vi "Temperature Engine Driver.vi"(11 "Sequence":refnum<k7>) -> (0 "error out":errorcluster)   [LabVIEW 2023, in "LTT_TeststandSteptypes.lvlib"]
uses:
  LTT_TeststandSteptypes.lvlib
  HardwareAbstractionLayer_LVOOP/Modbus/Modbus_class/Modbus.lvclass
  HardwareAbstractionLayer_LVOOP/Report/Report_class/Control/Temperature LOG.ctl
  Control/TC FGV Action.ctl
  HardwareAbstractionLayer_LVOOP/Power Moniter/Wait Monitor_class/SubVI/Control/TimerStates.ctl
  HardwareAbstractionLayer_LVOOP/Report/Report_class/Control/All Log Details.ctl
  HardwareAbstractionLayer_LVOOP/Report/Report_class/Control/UUT Test Info.ctl
  HardwareAbstractionLayer_LVOOP/Report/Report_class/Control/FE FRAME LOG.ctl
  HardwareAbstractionLayer_LVOOP/Report/Report_class/Control/FF FRAME LOG.ctl
  HardwareAbstractionLayer_LVOOP/Report/Report_class/Control/LIMIT TABLE.ctl
  HardwareAbstractionLayer_LVOOP/Report/Report_class/Control/ERROR LOG APPEND.ctl
  HardwareAbstractionLayer_LVOOP/Report/Report_class/Control/ERROR LOG.ctl
  HardwareAbstractionLayer_LVOOP/Report/Report_class/Control/FA FRAME LOG.ctl
  HardwareAbstractionLayer_LVOOP/Report/Report_class/Control/TEST RESULT LOG APPEND.ctl
  HardwareAbstractionLayer_LVOOP/Report/Report_class/Control/TEST RESULT LOG.ctl
  HardwareAbstractionLayer_LVOOP/Report/Report_class/Control/SYSTEM LOG.ctl
  HardwareAbstractionLayer_LVOOP/Report/Report_class/Control/POWER STATUS.ctl
  HardwareAbstractionLayer_LVOOP/Report/Report_class/Control/CYCLE_DURATION_LOG.ctl
  99722fe1-a764-4b52-b67b-c7e93846cf84.vi
  930c386e-a8bd-4bc2-a3c6-04cbbef34728.vi
  767a7da0-b67a-495a-b36e-4f64d8e2d20e.vi
  <vilib>/addons/TestStand/_TSUtility.llb/TestStand - Get Property Value (Boolean).vi
  GlobalVariable/GlobalVariableData.vi
  <vilib>/addons/TestStand/_TSUtility.llb/TestStand - Get Property Value (Number {Unsigned 32-bit Integer}).vi
  <vilib>/addons/TestStand/_TSUtility.llb/TestStand - Set Property Value (Number {Signed 16-bit Integer}).vi
  <vilib>/addons/TestStand/_TSUtility.llb/TestStand - Set Property Value (Boolean).vi
  <vilib>/addons/TestStand/_TSUtility.llb/TestStand - Set Property Value (String).vi
  HardwareAbstractionLayer_LVOOP/Database/Database.lvclass
  HardwareAbstractionLayer_LVOOP/Database/SQL Public VI/Control/DB Options.ctl
  HardwareAbstractionLayer_LVOOP/Teststand/Teststand.lvclass
  HardwareAbstractionLayer_LVOOP/Power Moniter/Wait Monitor_class/Wait Monitor.lvclass
  HardwareAbstractionLayer_LVOOP/Report/Report_class/Report.lvclass
panel:
  out "Array":i32[](array[numeric])
  out "End":string
  in  "Stop":bool
  in  "Modbus RTU":T1={"unit ID"=1, "serial type"=enum."RTU", "baud rate"=9600, "parity (even)"=2, "flow control (none)"=0, "VISA resource name"=""} {"flow control (none)" items=["None", "XON/XOFF", "RTS/CTS", "XON/XOFF & RTS/CTS", "DTR/DSR", "XON/XOFF & DTR/DSR"]; "parity (even)" items=["None", "Odd", "Even", "Mark", "Space"]}
  in  "error in":errorcluster
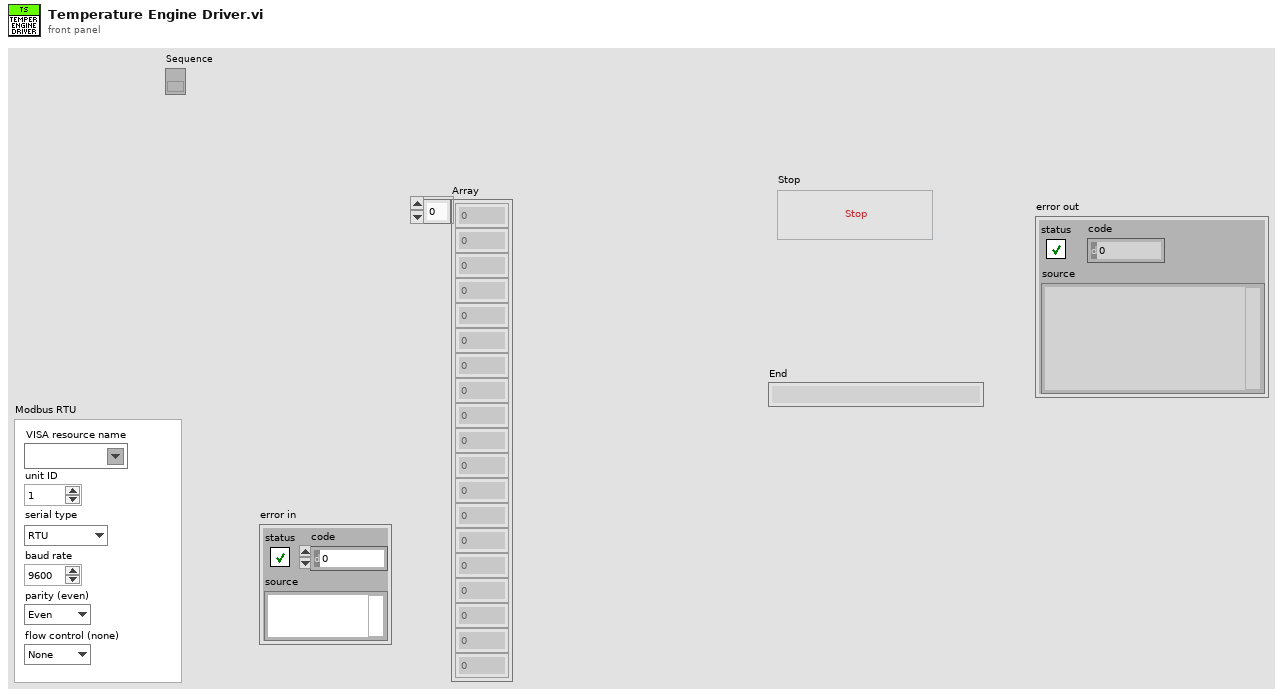
[diagram p1: front panel]
types:
  T1 = cluster{"unit ID":u8, "serial type":enum16{"RTU", "ASCII"}, "baud rate":u32, "parity (even)":u16, "flow control (none)":u16, "VISA resource name":refnum<visa-resource-name>}
  T2 = typedef "HardwareAbstractionLayer_LVOOP.lvlib/Report.lvclass/Temperature LOG.ctl" = cluster{"TEST_MODE":string, "CYCLE_NUMBER":string, "TEMPERATURE":cluster{"LV_PPS_TEMPERATURE":dbl, "HV_PPS1_TEMPERATURE":dbl, "HV_PPS2_TEMPERATURE":dbl, "HV_PPS3_TEMPERATURE":dbl, "HV_PPS4_TEMPERATURE":dbl, "HV_PPS5_TEMPERATURE":dbl, "HV_PPS6_TEMPERATURE":dbl, "CHAMBER_TEMPERATURE":dbl, "LOAD_U1_TEMPERATURE":dbl, "LOAD_V1_TEMPERATURE":dbl, "LOAD_W1_TEMPERATURE":dbl, "LOAD_U2_TEMPERATURE":dbl, "LOAD_V2_TEMPERATURE":dbl, "LOAD_W2_TEMPERATURE":dbl, "LOAD_U3_TEMPERATURE":dbl, "LOAD_V3_TEMPERATURE":dbl, "LOAD_W3_TEMPERATURE":dbl}, "Temperature Inrange":cluster{"LVPPS_Trip?":bool, "HVPPS1_Trip?":bool, "HVPPS2_Trip?":bool, "HVPPS3_Trip?":bool, "HVPPS4_Trip?":bool, "HVPPS5_Trip?":bool, "HVPPS6_Trip?":bool, "Chamber_Trip?":bool}}
  T3 = typedef "HardwareAbstractionLayer_LVOOP.lvlib/Database.lvclass/DB Options.ctl" = enum16{"Init", "Select Data", "Insert Data", "Update Data", "Delete Data", "Execute Query", "Create Schema", "Create Table", "List Tables", "List Columns", "Close"}
  T4 = typedef "TestStand - Status Monitor.ctl" = cluster{"Sequence Context":refnum<k7>, "Execution":refnum<k7>, "Termination Monitor":refnum<k7>}
  T5 = typedef "HardwareAbstractionLayer_LVOOP.lvlib/Report.lvclass/All Log Details.ctl" = cluster{"UUT_TEST_INFO":T6, "FE_FRAME_LOG":T7, "FF_FRAME_LOG":T8, "LIMIT_TABLE":T9, "ERROR LOG Append":T10, "FA_FRAME_LOG":T12, "Socket No":u16, "TEST RESULT LOG Append":T13, "SYSTEM_LOG":T15, "Temperature log":T2, "POWER_STATUS":T16, "CYCLE_DURATION_LOG":T17}
  T6 = typedef "HardwareAbstractionLayer_LVOOP.lvlib/Report.lvclass/UUT Test Info.ctl" = cluster{"ID":string, "STATION_ID":string, "TEST_SOCKET_INDEX":string, "UUT_SERIAL_NUMBER":string, "TSW_VER":string, "VAL_SW_VER":string, "PROJECT_NAME":string, "PRODUCT_NAME":string, "PRODUCT_VARIANT":string, "TEST_NAME":string, "TEST_PHASE":string, "TEST_DESCRIPTION":string, "TEMP_CHAMBER_NAME":string, "START_DATE_TIME":string, "STOP_DATE_TIME ":string, "START_CYCLE_COUNT":string, "STOP_CYCLE_COUNT":string, "EXECUTION_TIME":string, "UUT_STATUS":string, "UUT_ERROR_CODE":string, "UUT_ERROR_MESSAGE":string, "TEST_SEQUENCE":string}
  T7 = typedef "HardwareAbstractionLayer_LVOOP.lvlib/Report.lvclass/FE FRAME LOG.ctl" = cluster{"ID":string, "UUT_TEST_INFO":string, "DATE_TIME":string, "CYCLE_NUMBER":string, "TEST_MODE":string, "CHAMBER_TEMP":string, "CAN_FRAME_RX":string, "Test Mode":u32, "LV_PPS_VOLTAGE":string, "LV_PPS_CURRENT":string, "HV_PPS_VOLTAGE":string, "HV_PPS_CURRENT":string, "SOCKET_NUMBER":string, "CAN_FRAME_RX_NO_OFF_BYTE":string}
  T8 = typedef "HardwareAbstractionLayer_LVOOP.lvlib/Report.lvclass/FF FRAME LOG.ctl" = cluster{"ID":string, "UUT_TEST_INFO":string, "DATE_TIME":string, "CYCLE_NUMBER":string, "TEST_MODE":string, "CAN_FRAME_RX":string, "CHAMBER_TEMP":string, "TestMode":u32, "SOCKET_NUMBER":string, "CAN_FRAME_RX_NO_OFF_BYTE":string}
  T9 = typedef "HardwareAbstractionLayer_LVOOP.lvlib/Report.lvclass/LIMIT TABLE.ctl" = cluster{"ID":string, "PRODUCT_NAME":string, "PRODUCT_VARIANT":string, "TEST_MODE":string, "PARAMETER_NAME":string, "COMPARISON_TYPE":string, "LOW_LIMIT":string, "HIGH_LIMIT":string, "UNIT":string, "ERROR_MESSSAGE":string, "SEVERITY":string}
  T10 = typedef "HardwareAbstractionLayer_LVOOP.lvlib/Report.lvclass/ERROR LOG APPEND.ctl" = T11[]
  T11 = typedef "HardwareAbstractionLayer_LVOOP.lvlib/Report.lvclass/ERROR LOG.ctl" = cluster{"ID":string, "UUT_TEST_INFO":string, "DATE_TIME":string, "CYCLE_NUMBER":string, "TEST_MODE":string, "SIGNAL_NAME":string, "SIGNAL_VALUE":string, "UNIT":string, "COMPARISON_VALUE":string, "ERROR_MESSAGE":string, "FRAME_TYPE":string, "LIMITID":string, "SOCKET_NUMBER":string}
  T12 = typedef "HardwareAbstractionLayer_LVOOP.lvlib/Report.lvclass/FA FRAME LOG.ctl" = cluster{"UUT_TEST_INFO":string, "CAN_FRAME_RX":string, "CAN_FRAME_RX_NO_OFF_BYTE":string}
  T13 = typedef "HardwareAbstractionLayer_LVOOP.lvlib/Report.lvclass/TEST RESULT LOG APPEND.ctl" = T14[]
  T14 = typedef "HardwareAbstractionLayer_LVOOP.lvlib/Report.lvclass/TEST RESULT LOG.ctl" = cluster{"ID":string, "UUT_TEST_INFO":string, "DATE_TIME":string, "CYCLE_NUMBER":string, "TEST_MODE":string, "SIGNAL_NAME":string, "SIGNAL_VALUE":string, "COMPARISON_VALUE":string, "ERROR_MESSAGE":string, "FRAME_TYPE":string, "LIMITID":string, "TEST_RESULT":string, "SOCKET_NUMBER":string}
  T15 = typedef "HardwareAbstractionLayer_LVOOP.lvlib/Report.lvclass/SYSTEM LOG.ctl" = cluster{"ID ":string, "DATE_TIME":string, "CYCLE_NUMBER":string, "TEST_MODE":string, "ERROR_MESSAGE":string}
  T16 = typedef "HardwareAbstractionLayer_LVOOP.lvlib/Report.lvclass/POWER STATUS.ctl" = cluster{"TEST_MODE":string, "CYCLE_NUMBER":string, "TYPE_POWER":string, "STATE":string}
  T17 = typedef "HardwareAbstractionLayer_LVOOP.lvlib/Report.lvclass/CYCLE_DURATION_LOG.ctl" = cluster{"CYCLE_NUMBER":string}
  T18 = typedef "HardwareAbstractionLayer_LVOOP.lvlib/Wait Monitor.lvclass/TimerStates.ctl" = enum16{"Run", "Pause", "Reset"}
  T19 = typedef "LTT_TeststandSteptypes.lvlib/TC FGV Action.ctl" = enum16{"Set", "Get"}
  T20 = cluster{"Chamber Present Temp":dbl, "Chamber Target Temp":dbl, "Chamber RTD Temp":dbl}
  T21 = cluster{"LVPPS_Trip?":bool, "HVPPS1_Trip?":bool, "HVPPS2_Trip?":bool, "HVPPS3_Trip?":bool, "HVPPS4_Trip?":bool, "HVPPS5_Trip?":bool, "HVPPS6_Trip?":bool, "Chamber_Trip?":bool}
  T22 = cluster{"LV_PPS_TEMPERATURE":dbl, "HV_PPS1_TEMPERATURE":dbl, "HV_PPS2_TEMPERATURE":dbl, "HV_PPS3_TEMPERATURE":dbl, "HV_PPS4_TEMPERATURE":dbl, "HV_PPS5_TEMPERATURE":dbl, "HV_PPS6_TEMPERATURE":dbl, "CHAMBER_TEMPERATURE":dbl, "LOAD_U1_TEMPERATURE":dbl, "LOAD_V1_TEMPERATURE":dbl, "LOAD_W1_TEMPERATURE":dbl, "LOAD_U2_TEMPERATURE":dbl, "LOAD_V2_TEMPERATURE":dbl, "LOAD_W2_TEMPERATURE":dbl, "LOAD_U3_TEMPERATURE":dbl, "LOAD_V3_TEMPERATURE":dbl, "LOAD_W3_TEMPERATURE":dbl}
  T23 = typedef "HardwareAbstractionLayer_LVOOP.lvlib/Report.lvclass/Result FGV Data.ctl" = cluster{"Project Name":string, "Product Name":string, "Product Varient":string, "Test Name":string, "Test Phase":string, "Test Description":string, "Temp Chamber Name":string, "Schema":string, "Total No of Cycles":u32, "Current Cycle Number":u32, "Cycle Duration":u32, "Current Test Mode":string}
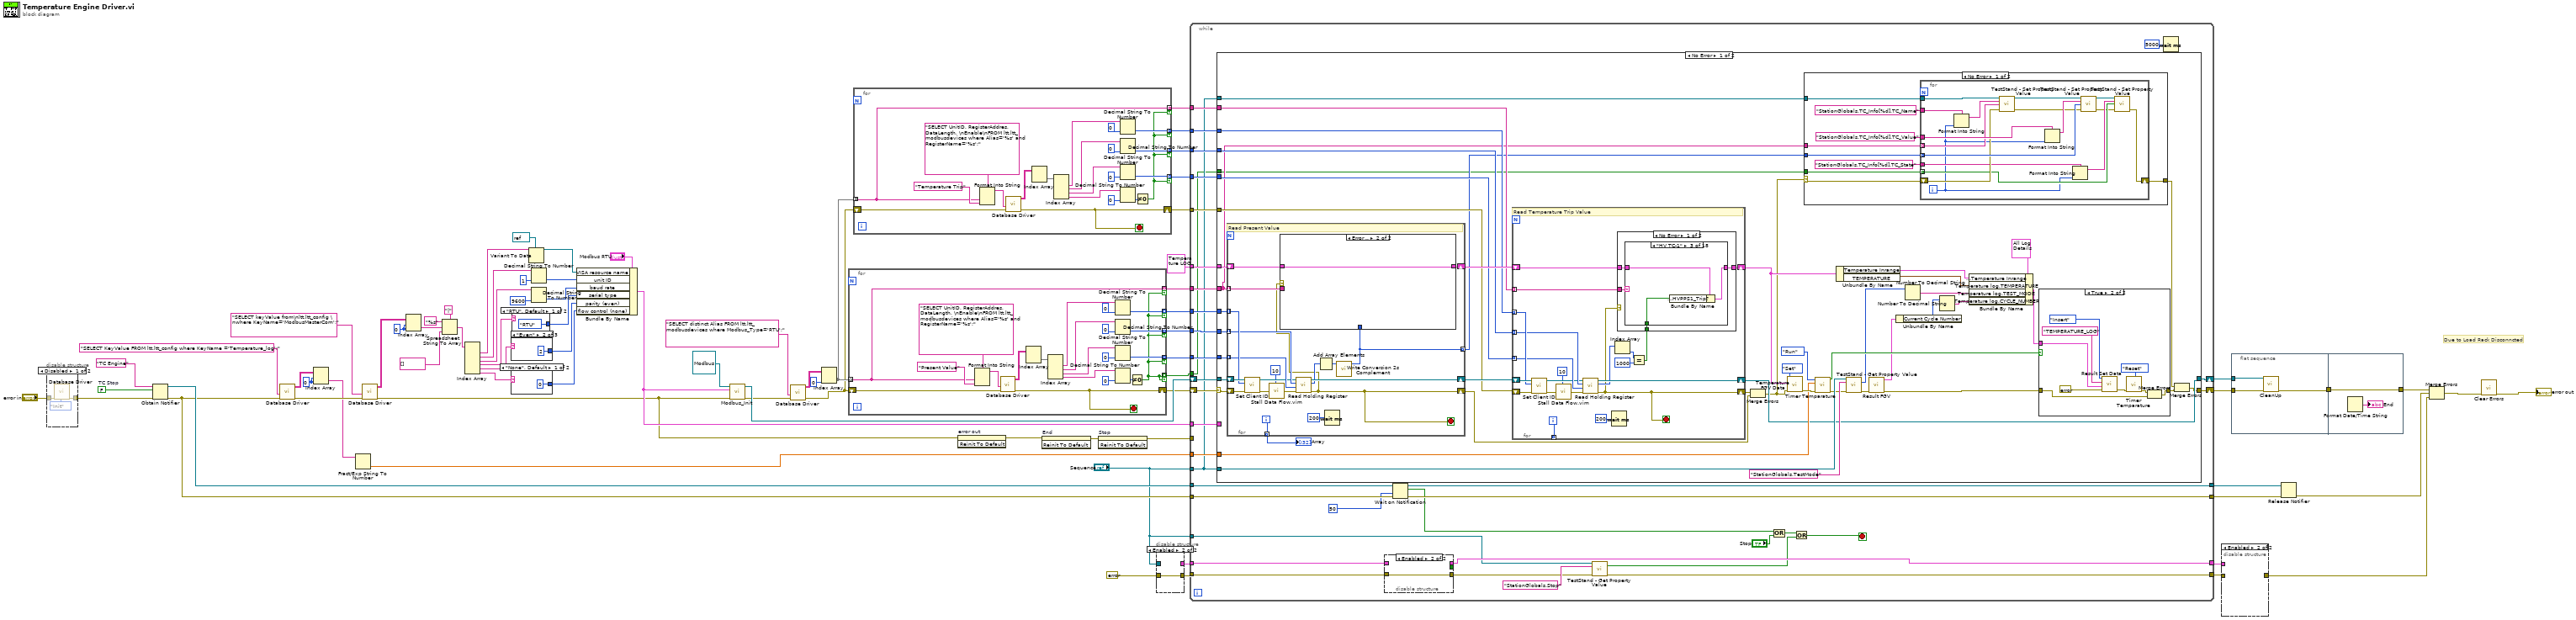
[diagram p0: block diagram]
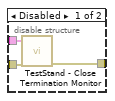
[diagram p2: hidden frame]
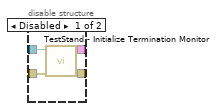
[diagram p3: hidden frame]
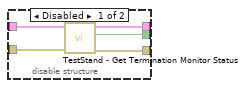
[diagram p5: hidden frame]
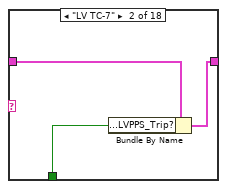
[diagram p8: hidden frame]
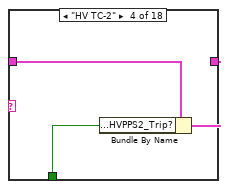
[diagram p9: hidden frame]
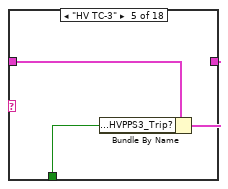
[diagram p10: hidden frame]
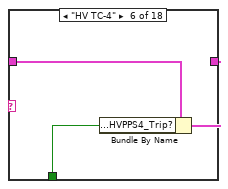
[diagram p11: hidden frame]
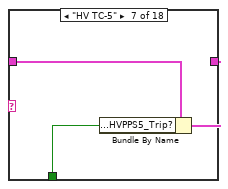
[diagram p12: hidden frame]
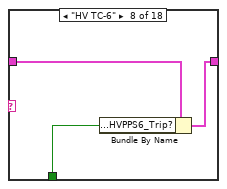
[diagram p13: hidden frame]
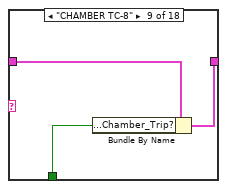
[diagram p14: hidden frame]
diagram:
  w19 = 0 ("disabled index (col)")
  w35 = FALSE  # TC Stop
  w74 = 0 ("index (row)")
  # "Due to Load Rack Disconncted"
  n1 = disable-structure shown="Disabled" {
    disable-tunnel: "error in" -> [w80 w81]
    disable-tunnel: [w79 w81] -> w34
    frame Disabled {
      n2 = call "Database Driver.vi"("Options"=DB_Options."Init", "error in"=w80) -> ("error out"=w79:errorcluster)  [unwired: 6 in, 3 out]
    }
    frame Enabled {
    }
  }
  n3 = Obtain Notifier(name (unnamed)="TC Engine", notification data type=w35, error in (no error)=w34) -> (notifier out=w33:refnum<notifier>, error out=w22:errorcluster)  [unwired: 1 in, 1 out]
  n4 = call "Database Driver.vi"("error in"=w22, "SQL query"="SELECT KeyValue FROM ltt.ltt_config where KeyName ='Temperature_log';" ("table")) -> ("error out"=w21:errorcluster, "data"=w20:string[][])  [unwired: 6 in, 2 out]
  n5 = Index Array(array=w20, index (row)=w19, index (col)=w19) -> (element=w18:string)
  n6 = Fract/Exp String To Number(string=w18) -> (number=w17:dbl)  [unwired: 3 in, 1 out]
  n7 = call "Database Driver.vi"("error in"=w21, "SQL query"="SELECT keyValue from\nltt.ltt_config \nwhere KeyName='ModbusMasterCom';") -> ("error out"=w26:errorcluster, "data"=w75:string[][])  [unwired: 6 in, 2 out]
  n8 = Index Array(array=w75, index (row)=w74, index (col)=w74) -> (element=w73:string)
  n9 = Spreadsheet String To Array(delimiter (Tab)="|" ("format string"), format string="%s", spreadsheet string=w73, array type (2D Dbl)=string[] []) -> (array=w71:string[])
  n10 = Index Array(array=w71) -> (element #1=w56:string, element #2=w69:string, element #3=w66:string, element #4=w63:string, element #5=w61:string, element #6=w60:string)  [unwired: 6 in]
  n11 = case shown="\"Even\"" w61 {
    tunnel: [u16 0 ("parity (even)") u16 2 ("parity (even)") u16 1 ("parity (even)")] -> w59
    frame "None", Default {
    }
    frame "Even" {
    }
    frame "Odd" {
    }
  }
  n12 = case shown="\"None\", Default" w60 {
    tunnel: [u16 0 ("flow control (none)") u16 1 ("flow control (none)")] -> w58
    frame "None", Default {
    }
    frame "True" {
    }
  }
  n13 = case shown="\"RTU\", Default" w63 {
    tunnel: [enum16{"RTU", "ASCII"}."RTU" ("serial type") enum16{"RTU", "ASCII"}."ASCII" ("serial type")] -> w62
    frame "RTU", Default {
    }
    frame "ASCII" {
    }
  }
  n14 = Variant To Data(type=refnum<visa-resource-name> refnum ("VISA resource name"), Variant=w56) -> (data=w55:refnum<visa-resource-name>)  [unwired: 1 in, 1 out]
  n15 = Decimal String To Number(string=w69, default (0L)=u8 1 ("unit ID")) -> (number=w67:u8)  [unwired: 1 in, 1 out]
  n16 = Decimal String To Number(string=w66, default (0L)=u32 9600 ("baud rate")) -> (number=w65:u32)  [unwired: 1 in, 1 out]
  n17 = Bundle By Name(cluster="Modbus RTU", "VISA resource name"=w55, "unit ID"=w67, "baud rate"=w65, "serial type"=w62, "parity (even)"=w59, "flow control (none)"=w58) -> (w27:T1)
  n18 = call "Modbus_Init.vi"("error in (no error)"=w26, "Modbus RTU"=w27, "object in"=refnum<class "Modbus.lvclass"> refnum ("VT_LTT.lvlib:Modbus")) -> ("error out"=w41:errorcluster, "object out"=w51:refnum<class "Modbus.lvclass">)  [unwired: 7 in]
  n19 = call "Database Driver.vi"("error in"=w41, "SQL query"="SELECT distinct Alias FROM ltt.ltt_modbusdevices where Modbus_Type='RTU';") -> ("error out"=w9:errorcluster, "data"=w42:string[][])  [unwired: 6 in, 2 out]
  n20 = Index Array(array=w42, index (col)=0 ("disabled index (col)")) -> (element=w10:string[])  [unwired: 1 in]
  n21 = for {
    tunnel: w10 -> [w90] mode=indexing
    tunnel: [w98] -> w39 mode=indexing if=w89
    tunnel: [w97] -> w38 mode=indexing if=w89
    tunnel: [w96] -> w37 mode=indexing if=w89
    shift-right: [w95] -> w40
    shift-left: w9 -> [w94]
    tunnel: [w90] -> w13 mode=indexing if=w89
    tunnel: [w89] -> w3 mode=indexing if=w89
    stop <- w95 stop-if-true
    n22 = Format Into String(format string="SELECT UnitID, RegisterAddres, DataLength, \nEnable\nFROM ltt.ltt_modbusdevices where Alias='%s' and RegisterName='%s';", w90, "Present Value" ("input 2")) -> (resulting string=w109:string)  [unwired: 2 in, 1 out]
    n23 = call "Database Driver.vi"("error in"=w94, "SQL query"=w109) -> ("error out"=w95:errorcluster, "data"=w108:string[][])  [unwired: 6 in, 2 out]
    n24 = Index Array(array=w108) -> (element=w107:string[])  [unwired: 2 in]
    n25 = Index Array(array=w107) -> (element #1=w106:string, element #2=w103:string, element #3=w102:string, element #4=w92:string)  [unwired: 4 in]
    n26 = Decimal String To Number(string=w106, default (0L)=u8 0 ("Slave unit ID")) -> (number=w98:u8)  [unwired: 1 in, 1 out]
    n27 = Decimal String To Number(string=w103, default (0L)=u16 0 ("starting address")) -> (number=w97:u16)  [unwired: 1 in, 1 out]
    n28 = Decimal String To Number(string=w102, default (0L)=u16 0 ("number of inputs")) -> (number=w96:u16)  [unwired: 1 in, 1 out]
    n29 = Decimal String To Number(string=w92, default (0L)=u16 0 ("number of inputs")) -> (number=w91:u16)  [unwired: 1 in, 1 out]
    n30 = Not Equal To 0?(x=w91) -> (x != 0?=w89:bool)
  }
  n31 = for {
    tunnel: w10 -> [w111] mode=indexing
    tunnel: [w119] -> w6 mode=indexing if=w110
    tunnel: [w118] -> w5 mode=indexing if=w110
    tunnel: [w117] -> w4 mode=indexing if=w110
    shift-right: [w116] -> w8
    shift-left: w9 -> [w115]
    tunnel: [w111] -> w7 mode=indexing if=w110
    stop <- w116 stop-if-true
    n32 = Format Into String(format string="SELECT UnitID, RegisterAddres, DataLength, \nEnable\nFROM ltt.ltt_modbusdevices where Alias='%s' and RegisterName='%s';", w111, "Temperature Trip" ("input 2")) -> (resulting string=w130:string)  [unwired: 2 in, 1 out]
    n33 = call "Database Driver.vi"("error in"=w115, "SQL query"=w130) -> ("error out"=w116:errorcluster, "data"=w129:string[][])  [unwired: 6 in, 2 out]
    n34 = Index Array(array=w129) -> (element=w128:string[])  [unwired: 2 in]
    n35 = Index Array(array=w128) -> (element #1=w127:string, element #2=w124:string, element #3=w123:string, element #4=w113:string)  [unwired: 4 in]
    n36 = Decimal String To Number(string=w127, default (0L)=u8 0 ("Slave unit ID")) -> (number=w119:u8)  [unwired: 1 in, 1 out]
    n37 = Decimal String To Number(string=w124, default (0L)=u16 0 ("starting address")) -> (number=w118:u16)  [unwired: 1 in, 1 out]
    n38 = Decimal String To Number(string=w123, default (0L)=u16 0 ("number of inputs")) -> (number=w117:u16)  [unwired: 1 in, 1 out]
    n39 = Decimal String To Number(string=w113, default (0L)=u16 0 ("number of inputs")) -> (number=w112:u16)  [unwired: 1 in, 1 out]
    n40 = Not Equal To 0?(x=w112) -> (x != 0?=w110:bool)
  }
  n41 = invoke on="error out" class="Clust (strict)" method="Reinit To Default"(error in=w26) -> (error out=w44:errorcluster)  [unwired: 2 in, 2 out]
  n42 = invoke on="End" class="Str" method="Reinit To Default"(error in=w44) -> (error out=w45:errorcluster)  [unwired: 2 in, 2 out]
  n43 = invoke on="Stop" class="Bool (strict)" method="Reinit To Default"(error in=w45) -> (error out=w46:errorcluster)  [unwired: 2 in, 2 out]
  n44 = disable-structure shown="Enabled" {
    disable-tunnel: [w134 _] -> w25
    disable-tunnel: [w133 w135] -> w24
    disable-tunnel: errorcluster {"status"=FALSE, "code"=0, "source"=""} ("error in (no error)") -> [w132 w135]
    disable-tunnel: "Sequence" -> [w131 _]
    frame Disabled {
      n45 = call <vilib>:"TestStand - Initialize Termination Monitor.vi"("error in (no error)"=w132, "Sequence Context In"=w131) -> ("error out"=w133:errorcluster, "Status Monitor Out"=w134:T4)  [unwired: 8 in]
    }
    frame Enabled {
    }
  }
  n46 = while {
    shift-right: [w167] -> w49
    shift-left: w40 -> [w171]
    shift-right: [w169] -> w50
    shift-left: w51 -> [w170]
    tunnel: w39 -> [w168]
    tunnel: w46 -> [_]
    tunnel: w38 -> [w166]
    tunnel: w37 -> [w165]
    tunnel: w33 -> [w164]
    tunnel: w22 -> [w163]
    tunnel: [w162] -> w32
    tunnel: [w161] -> w31
    tunnel: w27 -> [w152]
    tunnel: w25 -> [w160]
    tunnel: w24 -> [w159]
    tunnel: [w156] -> w23
    tunnel: w17 -> [w151]
    tunnel: w13 -> [w150]
    tunnel: T2 {"TEST_MODE"="", "CYCLE_NUMBER"="", "TEMPERATURE"={"LV_PPS_TEMPERATURE"=0.0, "HV_PPS1_TEMPERATURE"=0.0, "HV_PPS2_TEMPERATURE"=0.0, "HV_PPS3_TEMPERATURE"=0.0, "HV_PPS4_TEMPERATURE"=0.0, "HV_PPS5_TEMPERATURE"=0.0, "HV_PPS6_TEMPERATURE"=0.0, "CHAMBER_TEMPERATURE"=0.0, "LOAD_U1_TEMPERATURE"=0.0, "LOAD_V1_TEMPERATURE"=0.0, "LOAD_W1_TEMPERATURE"=0.0, "LOAD_U2_TEMPERATURE"=0.0, "LOAD_V2_TEMPERATURE"=0.0, "LOAD_W2_TEMPERATURE"=0.0, "LOAD_U3_TEMPERATURE"=0.0, "LOAD_V3_TEMPERATURE"=0.0, "LOAD_W3_TEMPERATURE"=0.0}, "Temperature Inrange"={"LVPPS_Trip?"=FALSE, "HVPPS1_Trip?"=FALSE, "HVPPS2_Trip?"=FALSE, "HVPPS3_Trip?"=FALSE, "HVPPS4_Trip?"=FALSE, "HVPPS5_Trip?"=FALSE, "HVPPS6_Trip?"=FALSE, "Chamber_Trip?"=FALSE}} ("Temperature log") -> [w149]
    tunnel: "Sequence" -> [w142]
    tunnel: w8 -> [w147]
    tunnel: w7 -> [w146]
    tunnel: w6 -> [w145]
    tunnel: w5 -> [w144]
    tunnel: w4 -> [w143]
    tunnel: w3 -> [w141]
    tunnel: "Sequence" -> [w139]
    tunnel: [w137] -> w1
    stop <- w158 stop-if-true
    n47 = case shown="No Error" w171 {
      selector: w171 -> [w222 w398]
      tunnel: w170 -> [w221 w401]
      tunnel: [w194 w403] -> w169
      tunnel: w168 -> [w220 _]
      tunnel: [w180 w404] -> w167
      tunnel: w166 -> [w219 _]
      tunnel: w165 -> [w218 _]
      tunnel: w152 -> [_ w405]
      tunnel: w151 -> [w212 _]
      tunnel: w150 -> [w183 _]
      tunnel: w149 -> [w210 _]
      tunnel: w142 -> [w204 _]
      tunnel: w147 -> [w190 _]
      tunnel: w146 -> [w185 _]
      tunnel: w145 -> [w193 _]
      tunnel: w144 -> [w192 _]
      tunnel: w143 -> [w191 _]
      tunnel: w142 -> [w184 _]
      tunnel: w141 -> [w178 _]
      frame No Error {
        n48 = for {
          tunnel: w220 -> [w334] mode=indexing
          shift-right: [w319] -> w188
          shift-left: w222 -> [w337]
          shift-right: [w335] -> w195
          shift-left: w221 -> [w336]
          tunnel: w219 -> [w332] mode=indexing
          tunnel: w218 -> [w331] mode=indexing
          tunnel: [w330] -> w211 mode=indexing
          tunnel: w183 -> [w323] mode=indexing
          shift-right: [w321] -> w197
          shift-left: w210 -> [w322]
          tunnel: [w320] -> w182 mode=indexing
          i -> [w330]
          stop <- w319 stop-if-true
          # "Read Present Value"
          n49 = call-dynamic "Set Client ID.vi"("error in (no error)"=w337, "Slave unit ID"=w334, "Modbus in"=w336) -> ("error out"=w329:errorcluster, "Modbus out"=w328:refnum<class "Modbus.lvclass">)  [unwired: 7 in]
          n50 = call "Stall Data Flow.vim"("value in"=w329, "milliseconds to wait"=u32 10) -> ("value out"=w327:errorcluster)  [unwired: 1 out]
          n51 = call-dynamic "Read Holding Register.vi"("error in (no error)"=w327, "number of inputs"=w331, "starting address"=w332, "Modbus in"=w328) -> ("error out"=w319:errorcluster, "register values"=w324:u16[], "Modbus out"=w335:refnum<class "Modbus.lvclass">)  [unwired: 5 in]
          n52 = Add Array Elements(numeric array=w324) -> (sum=w325:u16)
          n53 = Wait (ms)(milliseconds to wait=u32 200) -> ()  [unwired: 1 out]
          n54 = call "Write Conversion 2s Complement.vi"("Set Data Input"=w325) -> ("Coversion Data Output"=w320:i16)  [unwired: 10 in]
          n55 = case shown="Error .." w319 {
            tunnel: w323 -> [w341 _]
            tunnel: w322 -> [w340 w396]
            tunnel: [w339 w396] -> w321
            tunnel: w320 -> [w338 _]
            frame No Error {
              n56 = case shown="\"HV TC-6\"" w341 {
                tunnel: w340 -> [w342 w345 w348 w351 w354 w357 w360 w363 w368 w371 w374 w377 w380 w383 w386 w389 w392 w395]
                tunnel: [w342 w344 w347 w350 w353 w356 w359 w362 w367 w370 w373 w376 w379 w382 w385 w388 w391 w394] -> w339
                tunnel: w338 -> [_ w343 w346 w349 w352 w355 w358 w361 w365 w369 w372 w375 w378 w381 w384 w387 w390 w393]
                frame Default {
                }
                frame "LV TC-7" {
                  n57 = Bundle By Name(cluster=w345, "TEMPERATURE.LV_PPS_TEMPERATURE"=w343) -> (w344:T2)
                }
                frame "HV TC-1" {
                  n58 = Bundle By Name(cluster=w348, "TEMPERATURE.HV_PPS1_TEMPERATURE"=w346) -> (w347:T2)
                }
                frame "HV TC-2" {
                  n59 = Bundle By Name(cluster=w351, "TEMPERATURE.HV_PPS2_TEMPERATURE"=w349) -> (w350:T2)
                }
                frame "HV TC-3" {
                  n60 = Bundle By Name(cluster=w354, "TEMPERATURE.HV_PPS3_TEMPERATURE"=w352) -> (w353:T2)
                }
                frame "HV TC-4" {
                  n61 = Bundle By Name(cluster=w357, "TEMPERATURE.HV_PPS4_TEMPERATURE"=w355) -> (w356:T2)
                }
                frame "HV TC-5" {
                  n62 = Bundle By Name(cluster=w360, "TEMPERATURE.HV_PPS5_TEMPERATURE"=w358) -> (w359:T2)
                }
                frame "HV TC-6" {
                  n63 = Bundle By Name(cluster=w363, "TEMPERATURE.HV_PPS6_TEMPERATURE"=w361) -> (w362:T2)
                }
                frame "CHAMBER TC-8" {
                  # "Don't Forget Chamber Global Variable"
                  n64 = global read "GlobalVariableData.vi" "Chamber Temperature"() -> (w364:T20)
                  n65 = Bundle By Name(cluster=w364, "Chamber RTD Temp"=w365) -> (w366:T20)
                  n66 = global write "GlobalVariableData.vi" "Chamber Temperature"(w366) -> ()
                  n67 = Bundle By Name(cluster=w368, "TEMPERATURE.CHAMBER_TEMPERATURE"=w365) -> (w367:T2)
                }
                frame "LOAD TC-U1" {
                  n68 = Bundle By Name(cluster=w371, "TEMPERATURE.LOAD_U1_TEMPERATURE"=w369) -> (w370:T2)
                }
                frame "LOAD TC-V1" {
                  n69 = Bundle By Name(cluster=w374, "TEMPERATURE.LOAD_V1_TEMPERATURE"=w372) -> (w373:T2)
                }
                frame "LOAD TC-W1" {
                  n70 = Bundle By Name(cluster=w377, "TEMPERATURE.LOAD_W1_TEMPERATURE"=w375) -> (w376:T2)
                }
                frame "LOAD TC-U2" {
                  n71 = Bundle By Name(cluster=w380, "TEMPERATURE.LOAD_U2_TEMPERATURE"=w378) -> (w379:T2)
                }
                frame "LOAD TC-V2" {
                  n72 = Bundle By Name(cluster=w383, "TEMPERATURE.LOAD_V2_TEMPERATURE"=w381) -> (w382:T2)
                }
                frame "LOAD TC-W2" {
                  n73 = Bundle By Name(cluster=w386, "TEMPERATURE.LOAD_W2_TEMPERATURE"=w384) -> (w385:T2)
                }
                frame "LOAD TC-U3" {
                  n74 = Bundle By Name(cluster=w389, "TEMPERATURE.LOAD_U3_TEMPERATURE"=w387) -> (w388:T2)
                }
                frame "LOAD TC-V3" {
                  n75 = Bundle By Name(cluster=w392, "TEMPERATURE.LOAD_V3_TEMPERATURE"=w390) -> (w391:T2)
                }
                frame "LOAD TC-W3" {
                  n76 = Bundle By Name(cluster=w395, "TEMPERATURE.LOAD_W3_TEMPERATURE"=w393) -> (w394:T2)
                }
              }
            }
            frame Error {
            }
          }
        }
        "Array" <- w211
        n77 = for {
          tunnel: w193 -> [w266] mode=indexing
          shift-right: [w250] -> w189
          shift-left: w190 -> [w269]
          shift-right: [w267] -> w194
          shift-left: w195 -> [w268]
          tunnel: w192 -> [w264] mode=indexing
          tunnel: w191 -> [w263] mode=indexing
          tunnel: [w262] -> _ mode=indexing
          tunnel: w185 -> [w257] mode=indexing
          shift-right: [w255] -> w196
          shift-left: w197 -> [w256]
          i -> [w262]
          stop <- w250 stop-if-true
          # "Read Temperature Trip Value"
          n78 = call-dynamic "Set Client ID.vi"("error in (no error)"=w269, "Slave unit ID"=w266, "Modbus in"=w268) -> ("error out"=w261:errorcluster, "Modbus out"=w260:refnum<class "Modbus.lvclass">)  [unwired: 7 in]
          n79 = call "Stall Data Flow.vim"("value in"=w261, "milliseconds to wait"=u32 10) -> ("value out"=w259:errorcluster)  [unwired: 1 out]
          n80 = call-dynamic "Read Holding Register.vi"("error in (no error)"=w259, "number of inputs"=w263, "starting address"=w264, "Modbus in"=w260) -> ("error out"=w250:errorcluster, "register values"=w254:u16[], "Modbus out"=w267:refnum<class "Modbus.lvclass">)  [unwired: 5 in]
          n81 = Wait (ms)(milliseconds to wait=u32 200) -> ()  [unwired: 1 out]
          n82 = Index Array(array=w254) -> (element=w253:u16)  [unwired: 1 in]
          n83 = Equal?(x=w253, y=u16 1000) -> (x = y?=w251:bool)
          n84 = case shown="No Error" w250 {
            tunnel: w257 -> [w273 _]
            tunnel: w256 -> [w272 w308]
            tunnel: [w271 w308] -> w255
            tunnel: w251 -> [w270 _]
            frame No Error {
              n85 = case shown="\"HV TC-1\"" w273 {
                tunnel: w272 -> [w274 w277 w280 w283 w286 w289 w292 w295 w298 w299 w300 w301 w302 w303 w304 w305 w306 w307]
                tunnel: [w274 w276 w279 w282 w285 w288 w291 w294 w297 w299 w300 w301 w302 w303 w304 w305 w306 w307] -> w271
                tunnel: w270 -> [_ w275 w278 w281 w284 w287 w290 w293 w296 _ _ _ _ _ _ _ _ _]
                frame Default {
                }
                frame "LV TC-7" {
                  n86 = Bundle By Name(cluster=w277, "Temperature Inrange.LVPPS_Trip?"=w275) -> (w276:T2)
                }
                frame "HV TC-1" {
                  n87 = Bundle By Name(cluster=w280, "Temperature Inrange.HVPPS1_Trip?"=w278) -> (w279:T2)
                }
                frame "HV TC-2" {
                  n88 = Bundle By Name(cluster=w283, "Temperature Inrange.HVPPS2_Trip?"=w281) -> (w282:T2)
                }
                frame "HV TC-3" {
                  n89 = Bundle By Name(cluster=w286, "Temperature Inrange.HVPPS3_Trip?"=w284) -> (w285:T2)
                }
                frame "HV TC-4" {
                  n90 = Bundle By Name(cluster=w289, "Temperature Inrange.HVPPS4_Trip?"=w287) -> (w288:T2)
                }
                frame "HV TC-5" {
                  n91 = Bundle By Name(cluster=w292, "Temperature Inrange.HVPPS5_Trip?"=w290) -> (w291:T2)
                }
                frame "HV TC-6" {
                  n92 = Bundle By Name(cluster=w295, "Temperature Inrange.HVPPS6_Trip?"=w293) -> (w294:T2)
                }
                frame "CHAMBER TC-8" {
                  n93 = Bundle By Name(cluster=w298, "Temperature Inrange.Chamber_Trip?"=w296) -> (w297:T2)
                }
                frame "LOAD TC-U1" {
                }
                frame "LOAD TC-V1" {
                }
                frame "LOAD TC-W1" {
                }
                frame "LOAD TC-U2" {
                }
                frame "LOAD TC-V2" {
                }
                frame "LOAD TC-W2" {
                }
                frame "LOAD TC-U3" {
                }
                frame "LOAD TC-V3" {
                }
                frame "LOAD TC-W3" {
                }
              }
            }
            frame Error {
            }
          }
        }
        n94 = Merge Errors(w189, w188) -> (w181:errorcluster)
        n95 = call "Temperature FGV Data.vi"("error in"=w181, "Temperature log In"=w196, "Action"=TC_FGV_Action."Set") -> ("error out"=w216:errorcluster)  [unwired: 7 in, 1 out]
        n96 = case shown="No Error" w181 {
          selector: w181 -> [w226 w249]
          tunnel: w184 -> [w231 _]
          tunnel: w183 -> [w228 _]
          tunnel: w182 -> [w227 _]
          tunnel: [w225 w249] -> w179
          tunnel: w178 -> [w223 _]
          frame No Error {
            n97 = for {
              tunnel: w231 -> [w248]
              tunnel: "StationGlobals.TC_Info[%d].TC_Name" -> [w246]
              tunnel: "StationGlobals.TC_Info[%d].TC_Value" -> [w245]
              tunnel: w228 -> [w242] mode=indexing
              tunnel: w227 -> [w241] mode=indexing
              shift-right: [w234] -> w225
              shift-left: w226 -> [w240]
              tunnel: "StationGlobals.TC_Info[%d].TC_State" -> [w238]
              tunnel: w223 -> [w236] mode=indexing
              i -> [w232]
              n98 = Format Into String(format string=w246, w232) -> (resulting string=w247:string)  [unwired: 2 in, 1 out]
              n99 = call-poly <vilib>:"TestStand - Set Property Value.vi"("Sequence Context In"=w248, "Lookup String"=w247, "New Value"=w242, "error in (no error)"=w240) -> ("Sequence Context Out"=w244:refnum<k7>, "error out"=w239:errorcluster)  [unwired: 10 in]
              n100 = Format Into String(format string=w245, w232) -> (resulting string=w243:string)  [unwired: 2 in, 1 out]
              n101 = Format Into String(format string=w238, w232) -> (resulting string=w237:string)  [unwired: 2 in, 1 out]
              n102 = call-poly <vilib>:"TestStand - Set Property Value.vi"("Sequence Context In"=w244, "Lookup String"=w243, "New Value"=w241, "error in (no error)"=w239) -> ("Sequence Context Out"=w235:refnum<k7>, "error out"=w233:errorcluster)  [unwired: 10 in]
              n103 = call-poly <vilib>:"TestStand - Set Property Value.vi"("Sequence Context In"=w235, "Lookup String"=w237, "New Value"=w236, "error in (no error)"=w233) -> ("error out"=w234:errorcluster)  [unwired: 10 in, 1 out]
            }
          }
          frame Error {
          }
        }
        n104 = call "Timer Temparature.vi"("error in"=w216, "Set Time"=w212, "Options"=TimerStates."Run") -> ("error out"=w203:errorcluster, "Timeout?"=w213:bool)  [unwired: 5 in, 2 out]
        n105 = Unbundle By Name(w196) -> ("Temperature Inrange"=w187:T21, "TEMPERATURE"=w186:T22)
        n106 = call-poly <vilib>:"TestStand - Get Property Value.vi"("Sequence Context In"=w204, "Lookup String"="StationGlobals.TestMode", "error in (no error)"=w203) -> ("Value"=w201:u32, "error out"=w206:errorcluster)  [unwired: 10 in, 1 out]
        n107 = call "Result FGV.vi"("error in"=w206) -> ("error out"=w202:errorcluster, "Result FGV Data Out"=w207:T23)  [unwired: 9 in]
        n108 = Unbundle By Name(w207) -> ("Current Cycle Number"=w199:u32)
        n109 = Number To Decimal String(number=w201) -> (decimal integer string=w200:string)  [unwired: 1 in]
        n110 = Number To Decimal String(number=w199) -> (decimal integer string=w198:string)  [unwired: 1 in]
        n111 = Bundle By Name(cluster=T5 {"UUT_TEST_INFO"={"ID"="", "STATION_ID"="", "TEST_SOCKET_INDEX"="", "UUT_SERIAL_NUMBER"="", "TSW_VER"="", "VAL_SW_VER"="", "PROJECT_NAME"="", "PRODUCT_NAME"="", "PRODUCT_VARIANT"="", "TEST_NAME"="", "TEST_PHASE"="", "TEST_DESCRIPTION"="", "TEMP_CHAMBER_NAME"="", "START_DATE_TIME"="", "STOP_DATE_TIME "="", "START_CYCLE_COUNT"="", "STOP_CYCLE_COUNT"="", "EXECUTION_TIME"="", "UUT_STATUS"="", "UUT_ERROR_CODE"="", "UUT_ERROR_MESSAGE"="", "TEST_SEQUENCE"=""}, "FE_FRAME_LOG"={"ID"="", "UUT_TEST_INFO"="", "DATE_TIME"="", "CYCLE_NUMBER"="", "TEST_MODE"="", "CHAMBER_TEMP"="", "CAN_FRAME_RX"="", "Test Mode"=0, "LV_PPS_VOLTAGE"="", "LV_PPS_CURRENT"="", "HV_PPS_VOLTAGE"="", "HV_PPS_CURRENT"="", "SOCKET_NUMBER"="", "CAN_FRAME_RX_NO_OFF_BYTE"=""}, "FF_FRAME_LOG"={"ID"="", "UUT_TEST_INFO"="", "DATE_TIME"="", "CYCLE_NUMBER"="", "TEST_MODE"="", "CAN_FRAME_RX"="", "CHAMBER_TEMP"="", "TestMode"=0, "SOCKET_NUMBER"="", "CAN_FRAME_RX_NO_OFF_BYTE"=""}, "LIMIT_TABLE"={"ID"="", "PRODUCT_NAME"="", "PRODUCT_VARIANT"="", "TEST_MODE"="", "PARAMETER_NAME"="", "COMPARISON_TYPE"="", "LOW_LIMIT"="", "HIGH_LIMIT"="", "UNIT"="", "ERROR_MESSSAGE"="", "SEVERITY"=""}, "ERROR LOG Append"=[], "FA_FRAME_LOG"={"UUT_TEST_INFO"="", "CAN_FRAME_RX"="", "CAN_FRAME_RX_NO_OFF_BYTE"=""}, "Socket No"=1, "TEST RESULT LOG Append"=[], "SYSTEM_LOG"={"ID "="", "DATE_TIME"="", "CYCLE_NUMBER"="", "TEST_MODE"="", "ERROR_MESSAGE"=""}, "Temperature log"={"TEST_MODE"="", "CYCLE_NUMBER"="", "TEMPERATURE"={"LV_PPS_TEMPERATURE"=0.0, "HV_PPS1_TEMPERATURE"=0.0, "HV_PPS2_TEMPERATURE"=0.0, "HV_PPS3_TEMPERATURE"=0.0, "HV_PPS4_TEMPERATURE"=0.0, "HV_PPS5_TEMPERATURE"=0.0, "HV_PPS6_TEMPERATURE"=0.0, "CHAMBER_TEMPERATURE"=0.0, "LOAD_U1_TEMPERATURE"=0.0, "LOAD_V1_TEMPERATURE"=0.0, "LOAD_W1_TEMPERATURE"=0.0, "LOAD_U2_TEMPERATURE"=0.0, "LOAD_V2_TEMPERATURE"=0.0, "LOAD_W2_TEMPERATURE"=0.0, "LOAD_U3_TEMPERATURE"=0.0, "LOAD_V3_TEMPERATURE"=0.0, "LOAD_W3_TEMPERATURE"=0.0}, "Temperature Inrange"={"LVPPS_Trip?"=FALSE, "HVPPS1_Trip?"=FALSE, "HVPPS2_Trip?"=FALSE, "HVPPS3_Trip?"=FALSE, "HVPPS4_Trip?"=FALSE, "HVPPS5_Trip?"=FALSE, "HVPPS6_Trip?"=FALSE, "Chamber_Trip?"=FALSE}}, "POWER_STATUS"={"TEST_MODE"="", "CYCLE_NUMBER"="", "TYPE_POWER"="", "STATE"=""}, "CYCLE_DURATION_LOG"={"CYCLE_NUMBER"=""}} ("Set Data"), "Temperature log.Temperature Inrange"=w187, "Temperature log.TEMPERATURE"=w186, "Temperature log.TEST_MODE"=w200, "Temperature log.CYCLE_NUMBER"=w198) -> (w208:T5)
        n112 = case shown="True" w213 {
          tunnel: w202 -> [w309 w312]
          tunnel: [w309 w310] -> w214
          tunnel: w208 -> [_ w314]
          frame False {
          }
          frame True {
            n113 = call "Result Set Data.vi"("error in"=errorcluster {"status"=FALSE, "code"=0, "source"=""}, "Set Data"=w314, "Table Name"="TEMPERATURE_LOG", "Action"=enum16{"Insert", "Update"}."Insert") -> ("error out"=w316:errorcluster)  [unwired: 7 in]
            n114 = call "Timer Temparature.vi"("error in"=w316, "Options"=TimerStates."Reset") -> ("error out"=w311:errorcluster)  [unwired: 6 in, 3 out]
            n115 = Merge Errors(w311, w312) -> (w310:errorcluster)
          }
        }
        n116 = Merge Errors(w179, w214) -> (w180:errorcluster)
      }
      frame Error {
        n117 = call "PDU Status.vi"("error in"=errorcluster {"status"=FALSE, "code"=0, "source"=""}) -> ("error out"=w399:errorcluster, "OK"=w402:bool)  [unwired: 7 in, 2 out]
        n118 = Merge Errors(w399, w398) -> (w397:errorcluster)
        n119 = case shown="True" w402 {
          tunnel: w405 -> [_ w412]
          tunnel: [w406 w411] -> w404
          tunnel: [w407 w410] -> w403
          tunnel: w397 -> [w406 w409]
          tunnel: w401 -> [w407 _]
          frame False {
          }
          frame True {
            n120 = call <vilib>:"Clear Errors.vi"("error in (no error)"=w409) -> ("error out"=w408:errorcluster)  [unwired: 5 in, 1 out]
            n121 = call "Stall Data Flow.vim"("value in"=w408, "milliseconds to wait"=u32 1000) -> ("value out"=w413:errorcluster)  [unwired: 1 out]
            n122 = call "Modbus_Init.vi"("error in (no error)"=w413, "Modbus RTU"=w412, "object in"=refnum<class "Modbus.lvclass"> refnum ("VT_LTT.lvlib:Modbus")) -> ("error out"=w411:errorcluster, "object out"=w410:refnum<class "Modbus.lvclass">)  [unwired: 7 in]
          }
        }
      }
    }
    n123 = disable-structure shown="Enabled" {
      disable-tunnel: w160 -> [w176 _]
      disable-tunnel: w159 -> [w175 w177]
      disable-tunnel: [w174 _] -> _
      disable-tunnel: [w173 _] -> w156
      disable-tunnel: [w172 w177] -> w138
      frame Disabled {
        n124 = call <vilib>:"TestStand - Get Termination Monitor Status.vi"("error in (no error)"=w175, "Status Monitor In"=w176) -> ("error out"=w172:errorcluster, "Terminating or Aborting"=w174:bool, "Status Monitor Out"=w173:T4)  [unwired: 7 in]
      }
      frame Enabled {
      }
    }
    n125 = Wait on Notification(notifier=w164, timeout in ms (-1)=50, error in (no error)=w163) -> (notifier out=w162:refnum<notifier>, notification=w153:bool, error out=w161:errorcluster)  [unwired: 1 in, 1 out]
    n126 = call-poly <vilib>:"TestStand - Get Property Value.vi"("Sequence Context In"=w139, "Lookup String"="StationGlobals.Stop", "error in (no error)"=w138) -> ("Value"=w136:bool, "error out"=w137:errorcluster)  [unwired: 10 in, 1 out]
    n127 = Or(x=w153, y="Stop") -> (x .or. y?=w157:bool)
    n128 = Or(x=w157, y=w136) -> (x .or. y?=w158:bool)
    n129 = Wait (ms)(milliseconds to wait=u32 5000) -> ()  [unwired: 1 out]
  }
  n130 = disable-structure shown="Enabled" {
    disable-tunnel: w1 -> [w418 _]
    disable-tunnel: w23 -> [w417 _]
    disable-tunnel: [w416 _] -> w14
    frame Disabled {
      n131 = call <vilib>:"TestStand - Close Termination Monitor.vi"("error in (no error)"=w418, "Status Monitor In"=w417) -> ("error out"=w416:errorcluster)  [unwired: 9 in]
    }
    frame Enabled {
    }
  }
  n132 = flat-sequence {
    tunnel: w50 -> [w421]
    tunnel: w49 -> [w420]
    tunnel: [w419] -> w47
    tunnel: [w423] -> w48
    tunnel: w47 -> [w423]
    frame #0 {
      n133 = call-dynamic "CleanUp.vi"("object in"=w421, "error in (no error)"=w420) -> ("error out"=w419:errorcluster)  [unwired: 16 in, 1 out]
    }
    frame #1 {
      n134 = Format Date/Time String() -> (date/time string=→"End":string)  [unwired: 3 in]
    }
  }
  n135 = Release Notifier(notifier=w32, error in (no error)=w31) -> (error out=w29:errorcluster)  [unwired: 1 in, 2 out]
  n136 = Merge Errors(w48, w29, w14) -> (w30:errorcluster)
  n137 = call <vilib>:"Clear Errors.vi"("error in (no error)"=w30) -> ("error out"=→"error out":errorcluster)  [unwired: 5 in, 1 out]
